vi "main v1.vi"() -> ()   [LabVIEW 2015]
uses:
  <vilib>/userdefined/High Color/IMAQdx.ctl
  <vilib>/vision/driver/NI_Vision_Acquisition_Software.lvlib
panel:
  out "XY Graph":cluster{"X":dbl, "Y":dbl}[](graph)
  out "Image Center Position:All Elements":cluster{"X":u32, "Y":u32}
  out "xc_green":dbl
  out "yc_green":dbl
  out "yc_red":dbl
  out "xc_red":dbl
  out "yc":dbl
  out "xc":dbl
  out "angle GREEN radian":dbl
  out "angle GREEN degree":dbl
  out "distance GREEN in cm":dbl
  out "angle RED radian":dbl
  out "angle RED degree":dbl
  out "distance RED in cm":dbl
  out "Original":T1(plugin-control)
  out "Green Landmark Detection":T1(plugin-control)
  in  "Green Landmark Position X":i32
  in  "Green Landmark Position Y":i32
  in  "Red Landmark Position Y":i32
  in  "Red Landmark Position X":i32
  out "Red ROI":T2
  out "Red Landmark Horizontal Side":i32
  out "Red Landmark Vertical Side":i32
  out "Red Landmark Center.Y":sgl
  out "Red Landmark Center.X":sgl
  out "Red Landmark Detection":T1(plugin-control)
  out "Number of Red Landmarks":i32
  out "Green ROI":T2
  out "Green Landmark Horizontal Side":i32
  out "Green Landmark Vertical Side":i32
  out "Green Landmark Center.Y":sgl
  out "Green Landmark Center.X":sgl
  out "Number of Green Landmarks":i32
  in  "stop":bool
  in  "Session In":T3
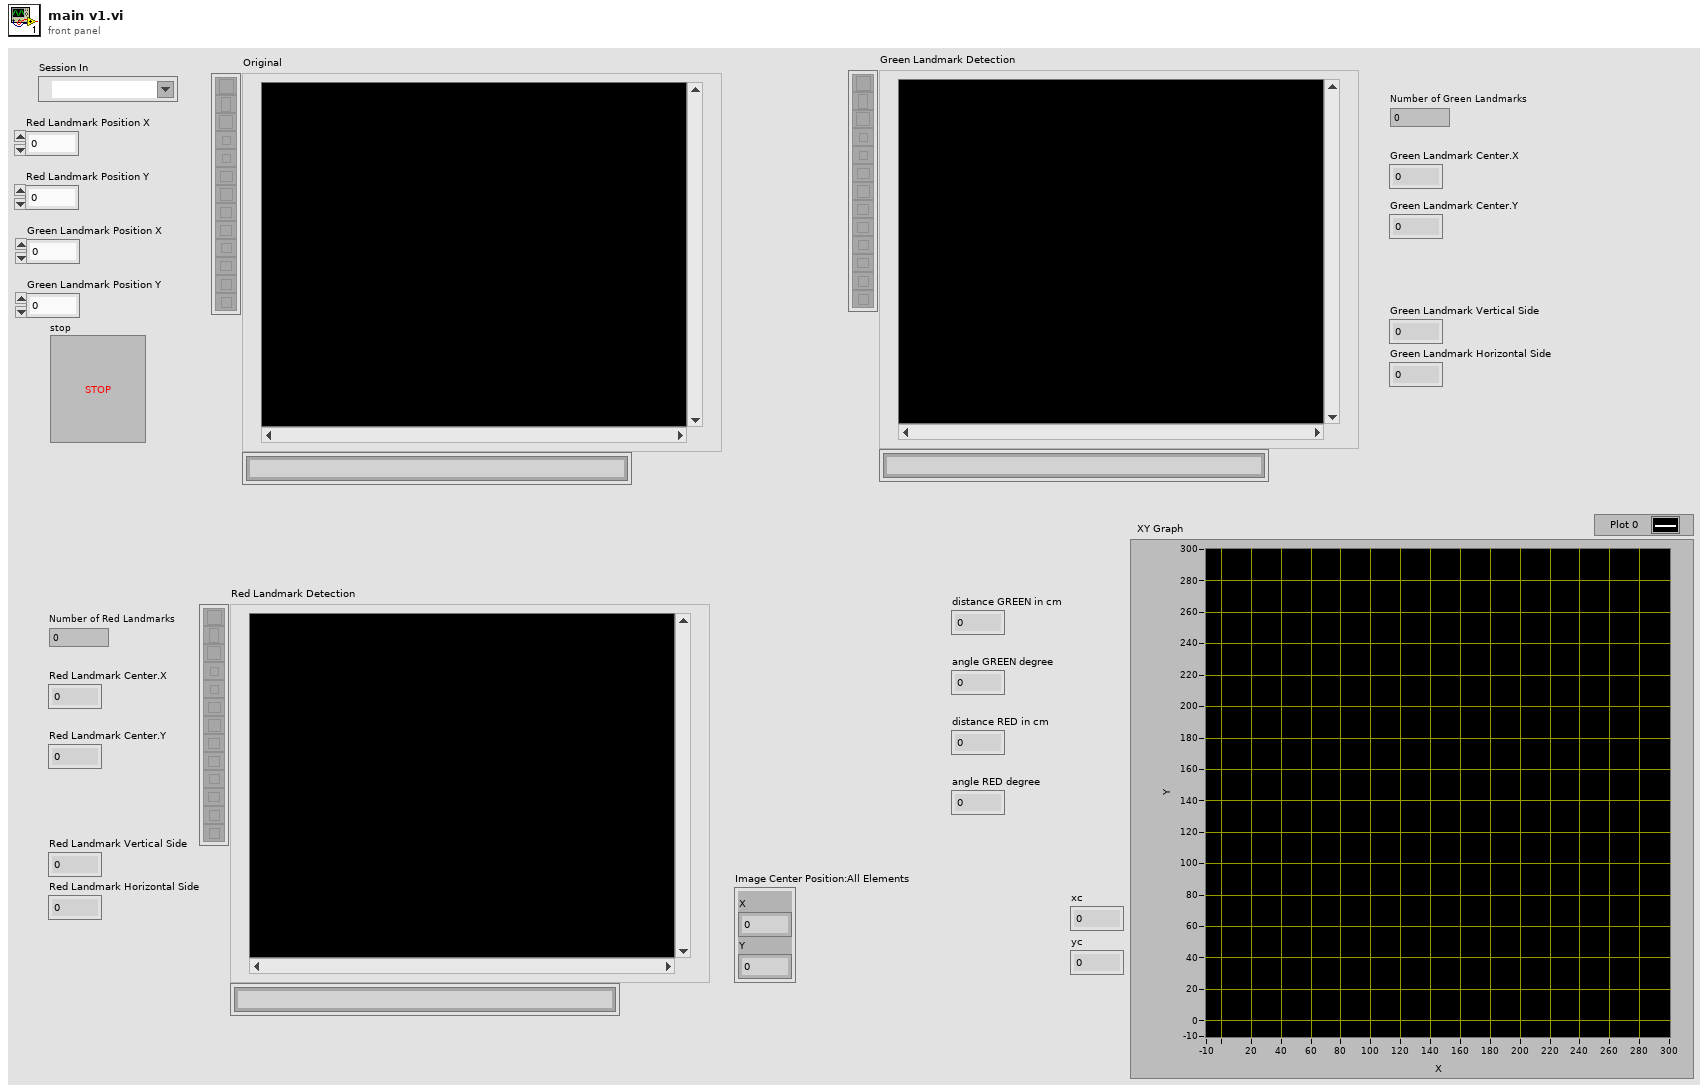
[diagram p1: front panel]
types:
  T1 = typedef "IMAQ Image.ctl" = refnum<image>
  T2 = cluster{"X Left":i32, "Y Top":i32, "X Right":i32, "Y Bottom":i32, "Rotation":i32}
  T3 = typedef "IMAQdx.ctl" = refnum<k21>
  T4 = typedef "Image Type" = u32
  T5 = enum16{"Landmark Detection", "ROI Landmark", "Red Landmark Distance calculation", "Green Landmark Distance calculation", "Camera Pose Estimation"}
  T6 = cluster{"Object Center":cluster{"X":sgl, "Y":sgl}, "Bounding Box":cluster{"X Left":i32, "Y Top":i32, "X Right":i32, "Y Bottom":i32}, "Area":sgl, "Orientation":sgl, "Aspect Ratio":sgl, "Nb Holes":i32}[]
  T7 = cluster{"Objects[0]":cluster{"Object Center":cluster{"X":sgl, "Y":sgl}, "Bounding Box":cluster{"X Left":i32, "Y Top":i32, "X Right":i32, "Y Bottom":i32}, "Area":sgl, "Orientation":sgl, "Aspect Ratio":sgl, "Nb Holes":i32}, "Objects[1]":cluster{"Object Center":cluster{"X":sgl, "Y":sgl}, "Bounding Box":cluster{"X Left":i32, "Y Top":i32, "X Right":i32, "Y Bottom":i32}, "Area":sgl, "Orientation":sgl, "Aspect Ratio":sgl, "Nb Holes":i32}, "Objects[2]":cluster{"Object Center":cluster{"X":sgl, "Y":sgl}, "Bounding Box":cluster{"X Left":i32, "Y Top":i32, "X Right":i32, "Y Bottom":i32}, "Area":sgl, "Orientation":sgl, "Aspect Ratio":sgl, "Nb Holes":i32}, "Objects[3]":cluster{"Object Center":cluster{"X":sgl, "Y":sgl}, "Bounding Box":cluster{"X Left":i32, "Y Top":i32, "X Right":i32, "Y Bottom":i32}, "Area":sgl, "Orientation":sgl, "Aspect Ratio":sgl, "Nb Holes":i32}, "Objects[4]":cluster{"Object Center":cluster{"X":sgl, "Y":sgl}, "Bounding Box":cluster{"X Left":i32, "Y Top":i32, "X Right":i32, "Y Bottom":i32}, "Area":sgl, "Orientation":sgl, "Aspect Ratio":sgl, "Nb Holes":i32}, "Objects[5]":cluster{"Object Center":cluster{"X":sgl, "Y":sgl}, "Bounding Box":cluster{"X Left":i32, "Y Top":i32, "X Right":i32, "Y Bottom":i32}, "Area":sgl, "Orientation":sgl, "Aspect Ratio":sgl, "Nb Holes":i32}, "Objects[6]":cluster{"Object Center":cluster{"X":sgl, "Y":sgl}, "Bounding Box":cluster{"X Left":i32, "Y Top":i32, "X Right":i32, "Y Bottom":i32}, "Area":sgl, "Orientation":sgl, "Aspect Ratio":sgl, "Nb Holes":i32}, "Objects[7]":cluster{"Object Center":cluster{"X":sgl, "Y":sgl}, "Bounding Box":cluster{"X Left":i32, "Y Top":i32, "X Right":i32, "Y Bottom":i32}, "Area":sgl, "Orientation":sgl, "Aspect Ratio":sgl, "Nb Holes":i32}, "Objects[8]":cluster{"Object Center":cluster{"X":sgl, "Y":sgl}, "Bounding Box":cluster{"X Left":i32, "Y Top":i32, "X Right":i32, "Y Bottom":i32}, "Area":sgl, "Orientation":sgl, "Aspect Ratio":sgl, "Nb Holes":i32}}
  T8 = cluster{"Object Center":cluster{"X":sgl, "Y":sgl}, "Bounding Box":cluster{"X Left":i32, "Y Top":i32, "X Right":i32, "Y Bottom":i32}, "Area":sgl, "Orientation":sgl, "Aspect Ratio":sgl, "Nb Holes":i32}
  T9 = cluster{"X Left":i32, "Y Top":i32, "X Right":i32, "Y Bottom":i32}
  T10 = typedef "ROI Descriptor" = cluster{"Global Rectangle":i32[], "Contours":cluster{"ID":enum32{"External", "Internal"}, "Type":u32, "Coordinates":i32[]}[]}
  T11 = cluster{"Green Landmark Position X":i32, "Green Landmark Position Y":i32}
  T12 = cluster{"Red Landmark Position X ":i32, "Red Landmark Position Y ":i32}
  T13 = cluster{"Green Landmark Position X":dbl, "Green Landmark Position Y":dbl}
  T14 = cluster{"Red Landmark Position X ":dbl, "Red Landmark Position Y ":dbl}
  T15 = cluster{"Red Landmark Position X ":dbl, "Red Landmark Position Y ":dbl}[]
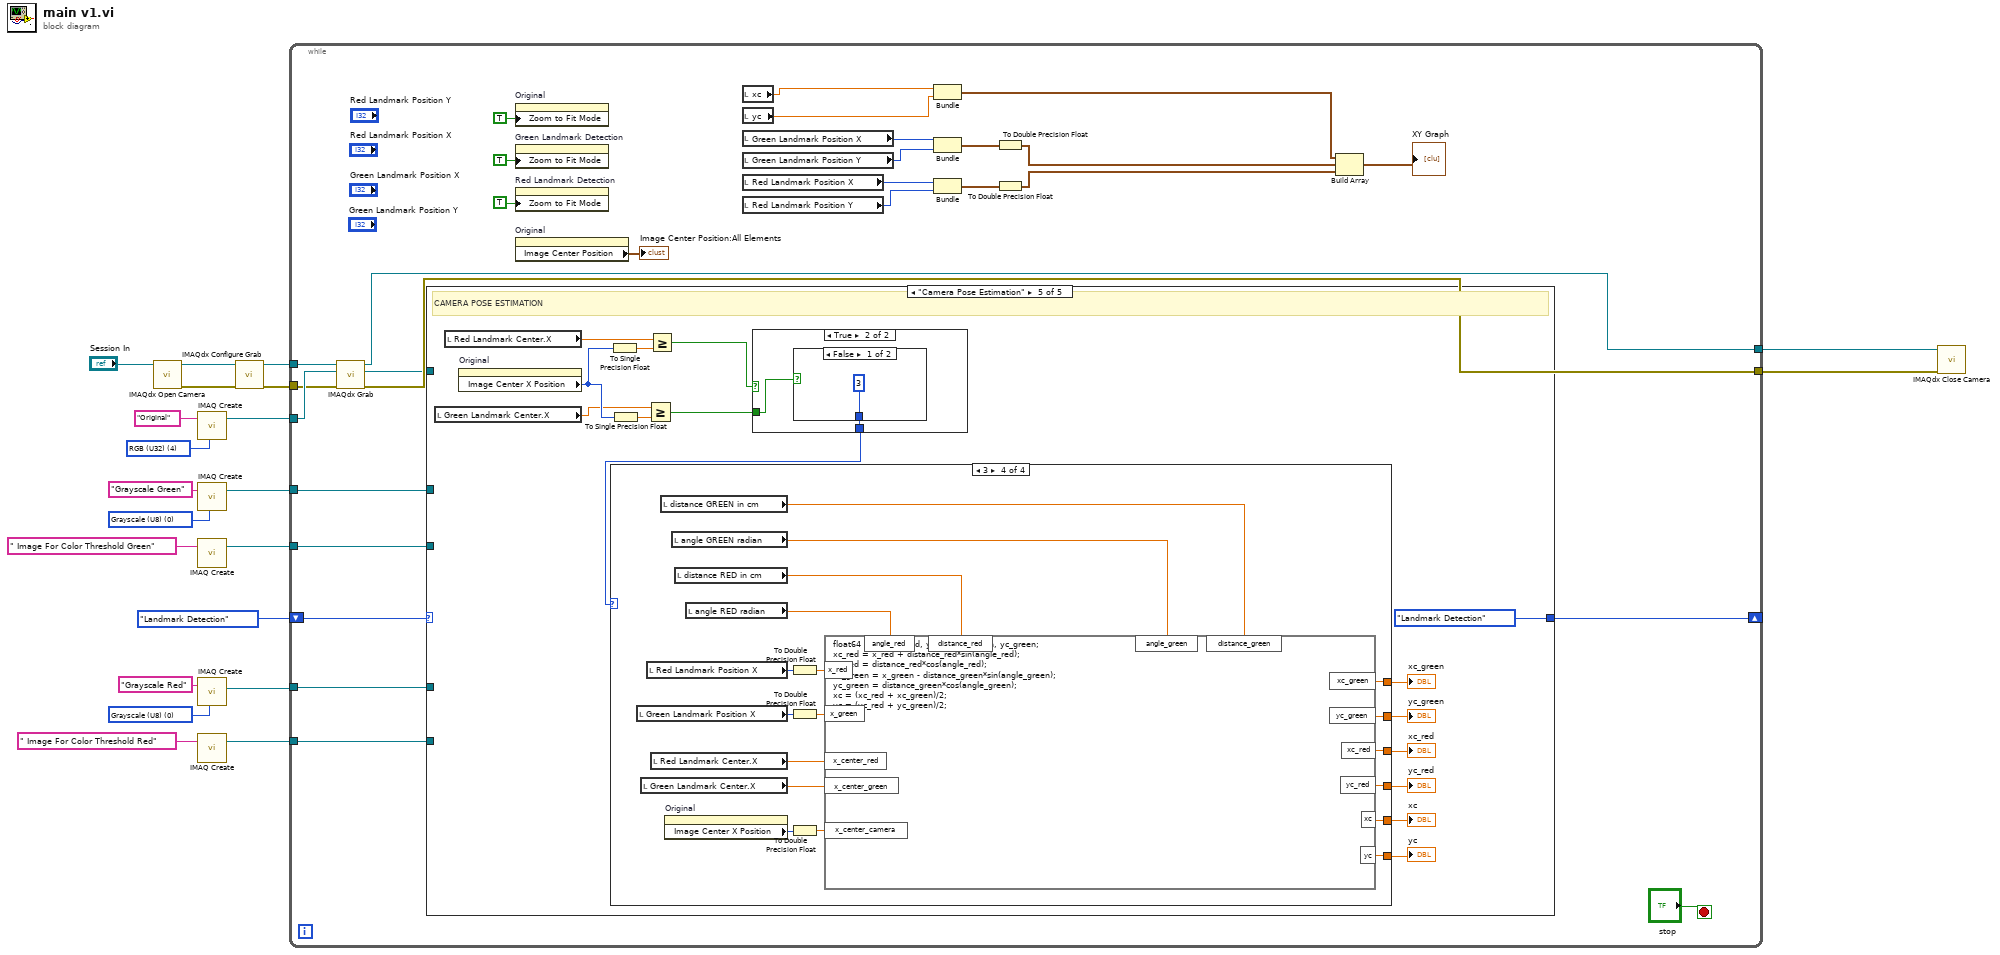
[diagram p0: block diagram]
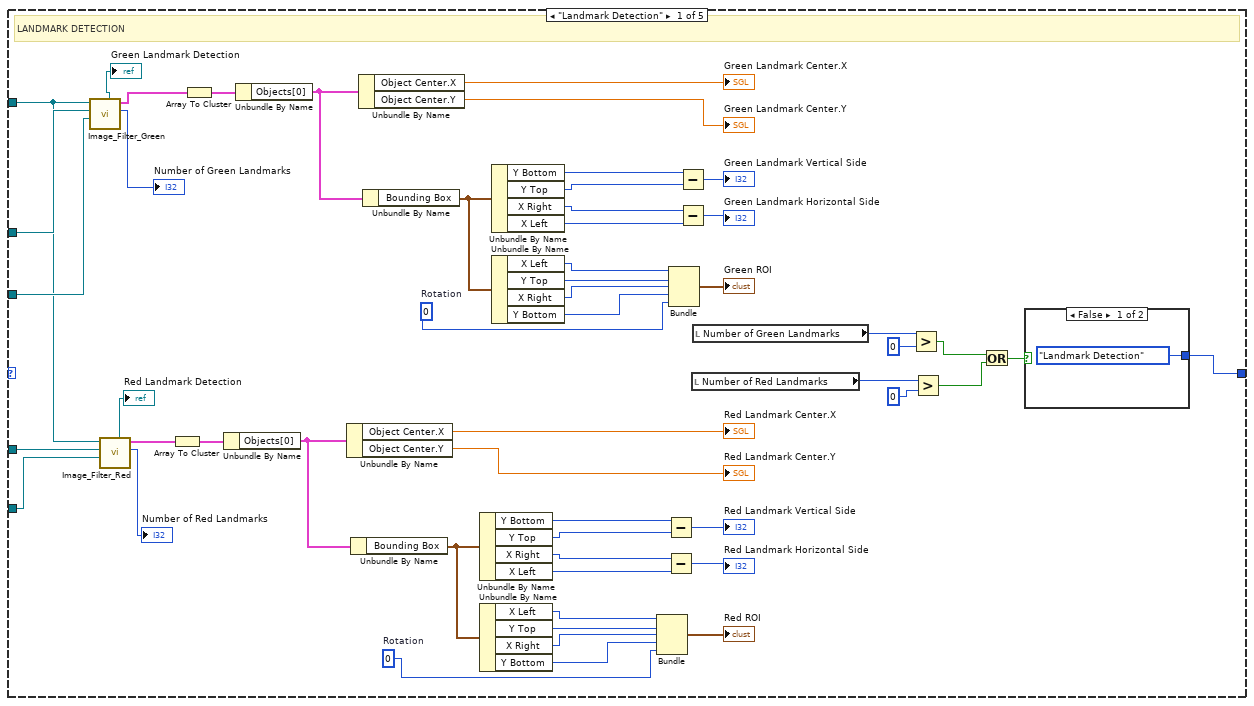
[diagram p2: hidden frame]
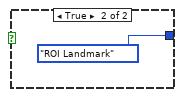
[diagram p3: hidden frame]
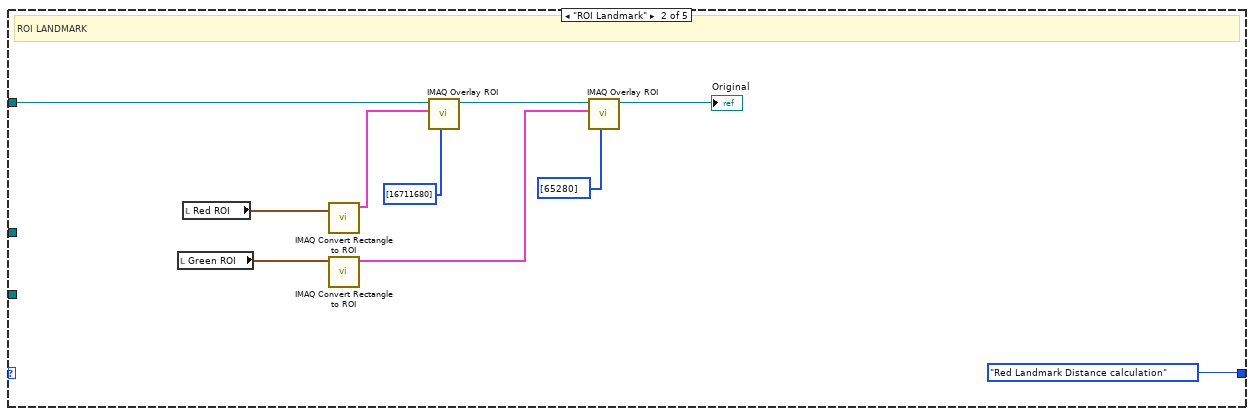
[diagram p4: hidden frame]
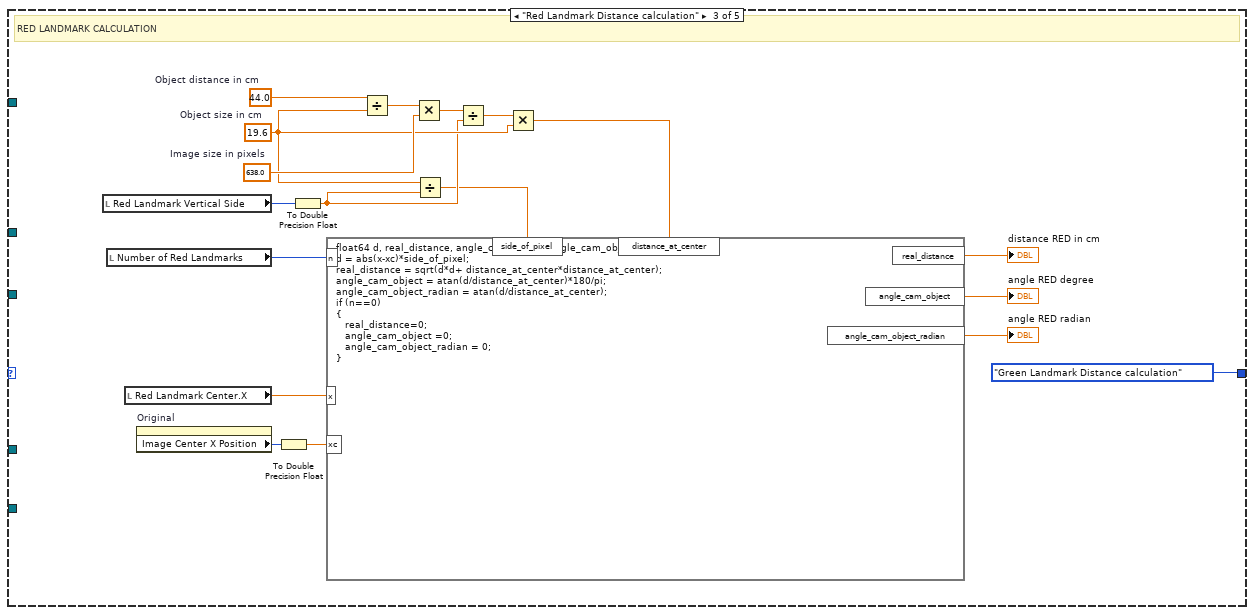
[diagram p5: hidden frame]
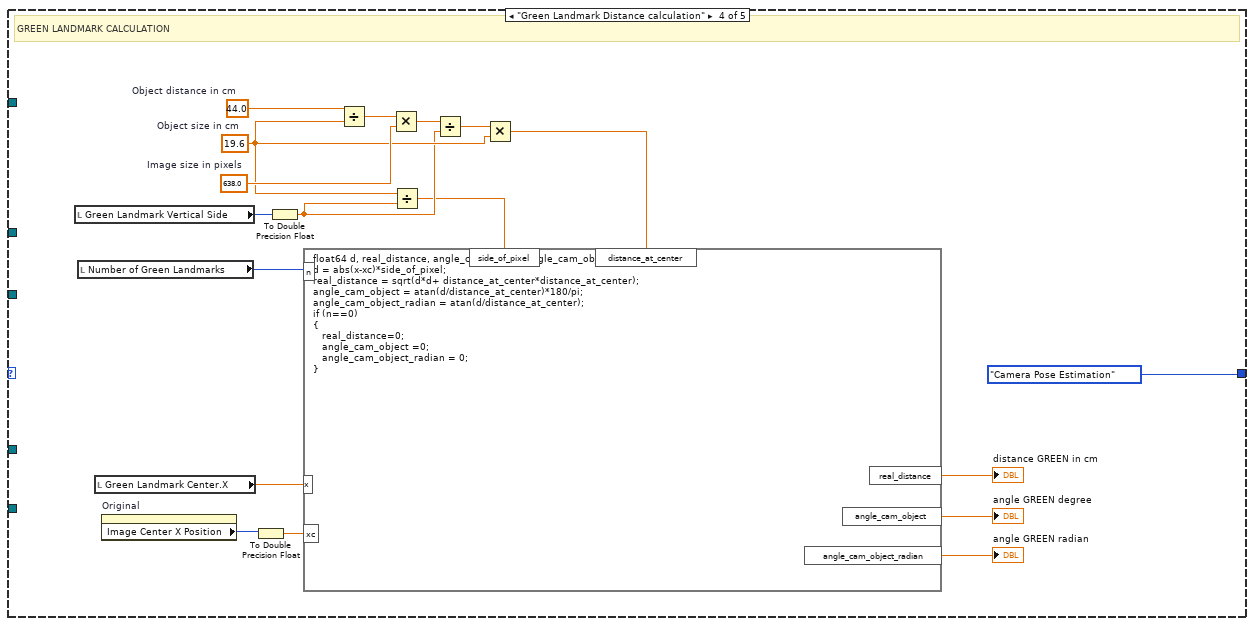
[diagram p6: hidden frame]
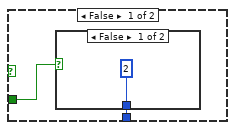
[diagram p7: hidden frame]
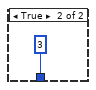
[diagram p8: hidden frame]
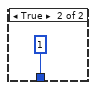
[diagram p9: hidden frame]
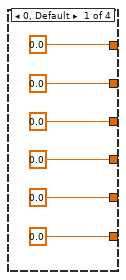
[diagram p10: hidden frame]
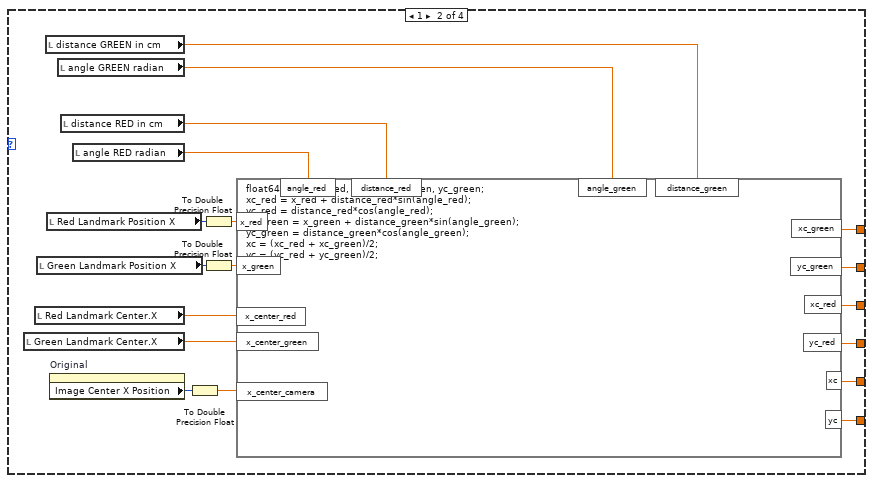
[diagram p11: hidden frame]
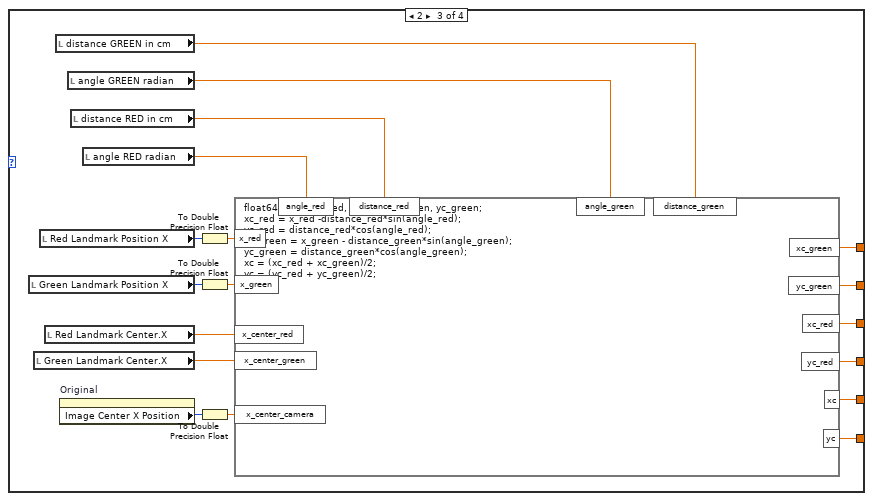
[diagram p12: hidden frame]
diagram:
  w4 = T4 0 items=["Grayscale (U8)", "Grayscale (I16)", "Grayscale (SGL)", "Complex (CSG)", "RGB (U32)", "HSL (U32)", "RGB (U64)", "Grayscale (U16)"] ("Image Type")
  w10 = T4 0 items=["Grayscale (U8)", "Grayscale (I16)", "Grayscale (SGL)", "Complex (CSG)", "RGB (U32)", "HSL (U32)", "RGB (U64)", "Grayscale (U16)"] ("Image Type")
  w14 = T4 4 items=["Grayscale (U8)", "Grayscale (I16)", "Grayscale (SGL)", "Complex (CSG)", "RGB (U32)", "HSL (U32)", "RGB (U64)", "Grayscale (U16)"] ("Image Type")
  n1 = call <vilib>:"IMAQdx Open Camera.vi"("Session In"="Session In") -> ("error out"=w18:errorcluster, "Session Out"=w21:T3)  [unwired: 9 in]
  n2 = call "IMAQ Create"("Image Name"="Original", "Image Type"=w14) -> ("New Image"=w17:T1)  [unwired: 3 in, 1 out]
  n3 = call "IMAQ Create"("Image Name"="Grayscale Green", "Image Type"=w10) -> ("New Image"=w8:T1)  [unwired: 3 in, 1 out]
  n4 = call "IMAQ Create"("Image Name"=" Image For Color Threshold Green") -> ("New Image"=w7:T1)  [unwired: 4 in, 1 out]
  n5 = call "IMAQ Create"("Image Name"="Grayscale Red", "Image Type"=w4) -> ("New Image"=w2:T1)  [unwired: 3 in, 1 out]
  n6 = call "IMAQ Create"("Image Name"=" Image For Color Threshold Red") -> ("New Image"=w1:T1)  [unwired: 4 in, 1 out]
  n7 = call <vilib>:"IMAQdx Configure Grab.vi"("error in"=w18, "Session In"=w21) -> ("error out"=w13:errorcluster, "Session Out"=w20:T3)  [unwired: 8 in]
  n8 = while {
    tunnel: w20 -> [w50]
    tunnel: w17 -> [w49]
    tunnel: [w43] -> w16
    tunnel: [w46] -> w15
    tunnel: w13 -> [w47]
    tunnel: w8 -> [w45]
    tunnel: w7 -> [w44]
    shift-right: [w38] -> _
    shift-left: T5."Landmark Detection" -> [w41]
    tunnel: w2 -> [w40]
    tunnel: w1 -> [w39]
    stop <- "stop" stop-if-true
    n9 = call <vilib>:"IMAQdx Grab.vi"("error in"=w47, "Image In"=w49, "Session In"=w50) -> ("error out"=w46:errorcluster, "Image Out"=w42:T1, "Session Out"=w43:T3)  [unwired: 5 in, 1 out]
    n10 = case shown="\"Camera Pose Estimation\"" w41 {
      tunnel: w45 -> [w86 _ _ _ _]
      tunnel: w44 -> [w85 _ _ _ _]
      tunnel: w42 -> [w62 w113 _ _ _]
      tunnel: w40 -> [w61 _ _ _ _]
      tunnel: w39 -> [w60 _ _ _ _]
      tunnel: [w52 T5."Red Landmark Distance calculation" T5."Green Landmark Distance calculation" T5."Camera Pose Estimation" T5."Landmark Detection"] -> w38
      frame "Landmark Detection" {
        w64 = 0  # Rotation
        w88 = 0  # Rotation
        # "LANDMARK DETECTION"
        n11 = call "Image_Filter_Green.vi"("Input Image"=w62, "New Image of IMAQ Threshold"=w86, "New Image for Color Threshold"=w85) -> ("Output Image of Object Detection"=→"Green Landmark Detection":T1, "Objects"=w83:T6, "Number of Objects"=→"Number of Green Landmarks":i32)  [unwired: 4 in]
        n12 = call "Image_Filter_Red.vi"("Input Image"=w62, "New Image of IMAQ Threshold"=w61, "New Image for Color Threshold"=w60) -> ("Output Image of Object Detection"=→"Red Landmark Detection":T1, "Objects"=w80:T6, "Number of Objects"=→"Number of Red Landmarks":i32)  [unwired: 4 in]
        n13 = Array To Cluster(array=w80) -> (cluster=w79:T7)
        n14 = Array To Cluster(array=w83) -> (cluster=w103:T7)
        n15 = Unbundle By Name(w79) -> ("Objects[0]"=w78:T8)
        n16 = Unbundle By Name(w103) -> ("Objects[0]"=w102:T8)
        n17 = Unbundle By Name(w78) -> ("Object Center.X"=→"Red Landmark Center.X":sgl, "Object Center.Y"=→"Red Landmark Center.Y":sgl)
        n18 = Unbundle By Name(w78) -> ("Bounding Box"=w69:T9)
        n19 = Unbundle By Name(w102) -> ("Object Center.X"=→"Green Landmark Center.X":sgl, "Object Center.Y"=→"Green Landmark Center.Y":sgl)
        n20 = Unbundle By Name(w102) -> ("Bounding Box"=w93:T9)
        n21 = Unbundle By Name(w69) -> ("Y Bottom"=w75:i32, "Y Top"=w74:i32, "X Right"=w73:i32, "X Left"=w72:i32)
        n22 = Unbundle By Name(w69) -> ("X Left"=w68:i32, "Y Top"=w67:i32, "X Right"=w66:i32, "Y Bottom"=w65:i32)
        n23 = Unbundle By Name(w93) -> ("Y Bottom"=w99:i32, "Y Top"=w98:i32, "X Right"=w97:i32, "X Left"=w96:i32)
        n24 = Unbundle By Name(w93) -> ("X Left"=w92:i32, "Y Top"=w91:i32, "X Right"=w90:i32, "Y Bottom"=w89:i32)
        n25 = Bundle("X Left"=w68, "Y Top"=w67, "X Right"=w66, "Y Bottom"=w65, "Rotation"=w64) -> (→"Red ROI":T2)  [unwired: 1 in]
        n26 = Subtract(x=w75, y=w74) -> (x-y=→"Red Landmark Vertical Side":i32)
        n27 = Subtract(x=w73, y=w72) -> (x-y=→"Red Landmark Horizontal Side":i32)
        n28 = Bundle("X Left"=w92, "Y Top"=w91, "X Right"=w90, "Y Bottom"=w89, "Rotation"=w88) -> (→"Green ROI":T2)  [unwired: 1 in]
        n29 = Subtract(x=w99, y=w98) -> (x-y=→"Green Landmark Vertical Side":i32)
        n30 = Subtract(x=w97, y=w96) -> (x-y=→"Green Landmark Horizontal Side":i32)
        n31 = local read "Number of Red Landmarks"() -> (w57:i32)
        n32 = local read "Number of Green Landmarks"() -> (w59:i32)
        n33 = Greater?(x=w59, y=0) -> (0:w55:bool)
        n34 = Greater?(x=w57, y=0) -> (0:w54:bool)
        n35 = Or(x=w55, y=w54) -> (x .or. y?=w53:bool)
        n36 = case shown="False" w53 {
          tunnel: [T5."Landmark Detection" T5."ROI Landmark"] -> w52
          frame False {
          }
          frame True {
          }
        }
      }
      frame "ROI Landmark" {
        # "ROI LANDMARK"
        n37 = local read "Green ROI"() -> (w114:T2)
        n38 = local read "Red ROI"() -> (w115:T2)
        n39 = call "IMAQ Convert Rectangle to ROI"("Rectangle"=w115) -> ("ROI Descriptor"=w112:T10)  [unwired: 8 in, 1 out]
        n40 = call "IMAQ Convert Rectangle to ROI"("Rectangle"=w114) -> ("ROI Descriptor"=w109:T10)  [unwired: 8 in, 1 out]
        n41 = call "IMAQ Overlay ROI"("Colors (Green)"=u32[] [16711680], "ROI Descriptor"=w112, "Image"=w113) -> ("Image Out"=w110:T1)  [unwired: 7 in, 1 out]
        n42 = call "IMAQ Overlay ROI"("Colors (Green)"=u32[] [65280], "ROI Descriptor"=w109, "Image"=w110) -> ("Image Out"=→"Original":T1)  [unwired: 7 in, 1 out]
      }
      frame "Red Landmark Distance calculation" {
        w127 = 638.0  # Image size in pixels
        w126 = 19.6  # Object size in cm
        w131 = 44.0  # Object distance in cm
        # "RED LANDMARK CALCULATION"
        n43 = local read "Red Landmark Vertical Side"() -> (w132:i32)
        n44 = local read "Number of Red Landmarks"() -> (w116:i32)
        n45 = local read "Red Landmark Center.X"() -> (w124:sgl)
        n46 = property on="Original" class="ImageControl"() -> ("Image Center X Position"=w123:u32)  [unwired: 2 in, 2 out]
        n47 = To Double Precision Float(number=w123) -> (double precision float=w122:dbl)
        n48 = To Double Precision Float(number=w132) -> (double precision float=w125:dbl)
        n49 = Divide(x=w131, y=w126) -> (x/y=w130:dbl)
        n50 = Multiply(x=w130, y=w127) -> (x*y=w128:dbl)
        n51 = Divide(x=w126, y=w125) -> (x/y=w120:dbl)
        n52 = Divide(x=w128, y=w125) -> (x/y=w129:dbl)
        n53 = Multiply(x=w129, y=w126) -> (x*y=w121:dbl)
        n54 = formula code="float64 d, real_distance, angle_cam_object, angle_cam_object_radian; \nd = abs(x-xc)*side_of_pixel;\nreal_distance = sqrt(d*d+ distance_at_center*distance_at_center);\nangle_cam_object = atan(d/distance_at_center)*180/pi;\nangle_cam_object_radian = atan(d/distance_at_center);\nif (n==0)\n{\n   real_distance=0;\n   angle_cam_object =0;\n   angle_cam_object_radian = 0;\n}"("x"=w124, "xc"=w122, "distance_at_center"=w121, "side_of_pixel"=w120, "n"=w116) -> ("real_distance"=→"distance RED in cm":dbl, "angle_cam_object"=→"angle RED degree":dbl, "angle_cam_object_radian"=→"angle RED radian":dbl)
      }
      frame "Green Landmark Distance calculation" {
        w145 = 638.0  # Image size in pixels
        w144 = 19.6  # Object size in cm
        w149 = 44.0  # Object distance in cm
        # "GREEN LANDMARK CALCULATION"
        n55 = local read "Green Landmark Vertical Side"() -> (w150:i32)
        n56 = local read "Number of Green Landmarks"() -> (w134:i32)
        n57 = local read "Green Landmark Center.X"() -> (w142:sgl)
        n58 = property on="Original" class="ImageControl"() -> ("Image Center X Position"=w135:u32)  [unwired: 2 in, 2 out]
        n59 = To Double Precision Float(number=w135) -> (double precision float=w141:dbl)
        n60 = To Double Precision Float(number=w150) -> (double precision float=w143:dbl)
        n61 = Divide(x=w149, y=w144) -> (x/y=w148:dbl)
        n62 = Multiply(x=w148, y=w145) -> (x*y=w146:dbl)
        n63 = Divide(x=w144, y=w143) -> (x/y=w139:dbl)
        n64 = Divide(x=w146, y=w143) -> (x/y=w147:dbl)
        n65 = Multiply(x=w147, y=w144) -> (x*y=w140:dbl)
        n66 = formula code="float64 d, real_distance, angle_cam_object, angle_cam_object_radian; \nd = abs(x-xc)*side_of_pixel;\nreal_distance = sqrt(d*d+ distance_at_center*distance_at_center);\nangle_cam_object = atan(d/distance_at_center)*180/pi;\nangle_cam_object_radian = atan(d/distance_at_center);\nif (n==0)\n{\n   real_distance=0;\n   angle_cam_object =0;\n   angle_cam_object_radian = 0;\n}"("x"=w142, "xc"=w141, "distance_at_center"=w140, "side_of_pixel"=w139, "n"=w134) -> ("real_distance"=→"distance GREEN in cm":dbl, "angle_cam_object"=→"angle GREEN degree":dbl, "angle_cam_object_radian"=→"angle GREEN radian":dbl)
      }
      frame "Camera Pose Estimation" {
        # "CAMERA POSE ESTIMATION"
        n67 = local read "Green Landmark Center.X"() -> (w154:sgl)
        n68 = local read "Red Landmark Center.X"() -> (w159:sgl)
        n69 = property on="Original" class="ImageControl"() -> ("Image Center X Position"=w157:u32)  [unwired: 2 in, 2 out]
        n70 = To Single Precision Float(number=w157) -> (single precision float=w158:sgl)
        n71 = To Single Precision Float(number=w157) -> (single precision float=w153:sgl)
        n72 = Greater Or Equal?(x=w154, y=w153) -> (x >= y?=w152:bool)
        n73 = Greater Or Equal?(x=w159, y=w158) -> (x >= y?=w156:bool)
        n74 = case shown="True" w156 {
          tunnel: [w168 w172] -> w155
          tunnel: w152 -> [w167 w171]
          frame False {
            n75 = case shown="False" w167 {
              tunnel: [2 3] -> w168
              frame False {
              }
              frame True {
              }
            }
          }
          frame True {
            n76 = case shown="False" w171 {
              tunnel: [3 1] -> w172
              frame False {
              }
              frame True {
              }
            }
          }
        }
        n77 = case shown="3" w155 {
          tunnel: [0.0 w190 w212 w230] -> w165
          tunnel: [0.0 w189 w211 w229] -> w164
          tunnel: [0.0 w188 w214 w232] -> w163
          tunnel: [0.0 w187 w213 w231] -> w162
          tunnel: [0.0 w186 w215 w233] -> w161
          tunnel: [0.0 w185 w216 w234] -> w160
          frame 0, Default {
          }
          frame 1 {
            n78 = local read "Green Landmark Center.X"() -> (w197:sgl)
            n79 = local read "Red Landmark Center.X"() -> (w198:sgl)
            n80 = local read "Green Landmark Position X"() -> (w184:i32)
            n81 = local read "distance GREEN in cm"() -> (w192:dbl)
            n82 = local read "Red Landmark Position X"() -> (w182:i32)
            n83 = property on="Original" class="ImageControl"() -> ("Image Center X Position"=w195:u32)  [unwired: 2 in, 2 out]
            n84 = local read "angle GREEN radian"() -> (w191:dbl)
            n85 = local read "distance RED in cm"() -> (w193:dbl)
            n86 = local read "angle RED radian"() -> (w194:dbl)
            n87 = To Double Precision Float(number=w195) -> (double precision float=w196:dbl)
            n88 = To Double Precision Float(number=w182) -> (double precision float=w181:dbl)
            n89 = To Double Precision Float(number=w184) -> (double precision float=w183:dbl)
            n90 = formula code="float64 xc, yc, xc_red, yc_red, xc_green, yc_green;\nxc_red = x_red + distance_red*sin(angle_red);\nyc_red = distance_red*cos(angle_red);\nxc_green = x_green + distance_green*sin(angle_green);\nyc_green = distance_green*cos(angle_green);\nxc = (xc_red + xc_green)/2; \nyc = (yc_red + yc_green)/2;"("x_center_red"=w198, "x_center_green"=w197, "x_center_camera"=w196, "angle_red"=w194, "angle_green"=w191, "distance_red"=w193, "distance_green"=w192, "x_red"=w181, "x_green"=w183) -> ("xc"=w190:dbl, "yc"=w189:dbl, "xc_red"=w188:dbl, "yc_red"=w187:dbl, "xc_green"=w185:dbl, "yc_green"=w186:dbl)
          }
          frame 2 {
            n91 = local read "Green Landmark Position X"() -> (w204:i32)
            n92 = local read "Green Landmark Center.X"() -> (w199:sgl)
            n93 = local read "Red Landmark Position X"() -> (w201:i32)
            n94 = local read "Red Landmark Center.X"() -> (w200:sgl)
            n95 = local read "distance GREEN in cm"() -> (w207:dbl)
            n96 = property on="Original" class="ImageControl"() -> ("Image Center X Position"=w206:u32)  [unwired: 2 in, 2 out]
            n97 = local read "angle GREEN radian"() -> (w208:dbl)
            n98 = local read "distance RED in cm"() -> (w209:dbl)
            n99 = local read "angle RED radian"() -> (w210:dbl)
            n100 = To Double Precision Float(number=w201) -> (double precision float=w202:dbl)
            n101 = To Double Precision Float(number=w204) -> (double precision float=w203:dbl)
            n102 = To Double Precision Float(number=w206) -> (double precision float=w205:dbl)
            n103 = formula code="float64 xc, yc, xc_red, yc_red, xc_green, yc_green;\nxc_red = x_red -distance_red*sin(angle_red);\nyc_red = distance_red*cos(angle_red);\nxc_green = x_green - distance_green*sin(angle_green);\nyc_green = distance_green*cos(angle_green);\nxc = (xc_red + xc_green)/2; \nyc = (yc_red + yc_green)/2;"("x_center_red"=w200, "x_center_green"=w199, "x_center_camera"=w205, "angle_red"=w210, "angle_green"=w208, "distance_red"=w209, "distance_green"=w207, "x_red"=w202, "x_green"=w203) -> ("xc"=w212:dbl, "yc"=w211:dbl, "xc_red"=w214:dbl, "yc_red"=w213:dbl, "xc_green"=w216:dbl, "yc_green"=w215:dbl)
          }
          frame 3 {
            n104 = local read "Green Landmark Position X"() -> (w222:i32)
            n105 = local read "Green Landmark Center.X"() -> (w219:sgl)
            n106 = local read "Red Landmark Position X"() -> (w224:i32)
            n107 = local read "Red Landmark Center.X"() -> (w220:sgl)
            n108 = local read "distance GREEN in cm"() -> (w225:dbl)
            n109 = property on="Original" class="ImageControl"() -> ("Image Center X Position"=w218:u32)  [unwired: 2 in, 2 out]
            n110 = local read "angle GREEN radian"() -> (w226:dbl)
            n111 = local read "distance RED in cm"() -> (w227:dbl)
            n112 = local read "angle RED radian"() -> (w228:dbl)
            n113 = To Double Precision Float(number=w224) -> (double precision float=w223:dbl)
            n114 = To Double Precision Float(number=w222) -> (double precision float=w221:dbl)
            n115 = To Double Precision Float(number=w218) -> (double precision float=w217:dbl)
            n116 = formula code="float64 xc, yc, xc_red, yc_red, xc_green, yc_green;\nxc_red = x_red + distance_red*sin(angle_red);\nyc_red = distance_red*cos(angle_red);\nxc_green = x_green - distance_green*sin(angle_green);\nyc_green = distance_green*cos(angle_green);\nxc = (xc_red + xc_green)/2; \nyc = (yc_red + yc_green)/2;"("x_center_red"=w220, "x_center_green"=w219, "x_center_camera"=w217, "angle_red"=w228, "angle_green"=w226, "distance_red"=w227, "distance_green"=w225, "x_red"=w223, "x_green"=w221) -> ("xc"=w230:dbl, "yc"=w229:dbl, "xc_red"=w232:dbl, "yc_red"=w231:dbl, "xc_green"=w234:dbl, "yc_green"=w233:dbl)
          }
        }
        "xc" <- w165
        "yc" <- w164
        "xc_red" <- w163
        "yc_red" <- w162
        "yc_green" <- w161
        "xc_green" <- w160
      }
    }
    n117 = property on="Original" class="ImageControl"("Zoom to Fit Mode"=TRUE) -> ()  [unwired: 2 in, 2 out]
    n118 = property on="Green Landmark Detection" class="ImageControl"("Zoom to Fit Mode"=TRUE) -> ()  [unwired: 2 in, 2 out]
    n119 = property on="Red Landmark Detection" class="ImageControl"("Zoom to Fit Mode"=TRUE) -> ()  [unwired: 2 in, 2 out]
    n120 = property on="Original" class="ImageControl"() -> ("Image Center Position"=→"Image Center Position:All Elements":cluster{"X":u32, "Y":u32})  [unwired: 2 in, 2 out]
    n121 = local read "xc"() -> (w24:dbl)
    n122 = local read "yc"() -> (w25:dbl)
    n123 = local read "Green Landmark Position X"() -> (w33:i32)
    n124 = local read "Green Landmark Position Y"() -> (w32:i32)
    n125 = local read "Red Landmark Position X"() -> (w22:i32)
    n126 = local read "Red Landmark Position Y"() -> (w23:i32)
    n127 = Bundle("xc"=w24, "yc"=w25) -> (w29:cluster{"xc":dbl, "yc":dbl})  [unwired: 1 in]
    n128 = Bundle("Green Landmark Position X"=w33, "Green Landmark Position Y"=w32) -> (w31:T11)  [unwired: 1 in]
    n129 = Bundle("Red Landmark Position X"=w22, "Red Landmark Position Y"=w23) -> (w30:T12)  [unwired: 1 in]
    n130 = To Double Precision Float(number=w31) -> (double precision float=w28:T13)
    n131 = To Double Precision Float(number=w30) -> (double precision float=w27:T14)
    n132 = Build Array(w29, w28, w27) -> (→"XY Graph":T15)
  }
  n133 = call <vilib>:"IMAQdx Close Camera.vi"("error in"=w15, "Session In"=w16) -> ()  [unwired: 9 in, 1 out]
